vi "main.vi"() -> ()   [LabVIEW 2022 SP3]
uses:
  <vilib>/express/express arith-compare/Formula/XNode/ExpressFormulaBlockNode.xnode
panel:
  in  "Día":i32=1 min=1 max=365
  out "Dia_a":i32
  out "Diciembre":bool
  out "Noviembre":bool
  out "Octubre":bool
  out "Septiembre":bool
  out "Agosto":bool
  out "Julio":bool
  out "Junio":bool
  out "Mayo":bool
  out "Abril":bool
  out "Marzo":bool
  out "Febrero":bool
  out "Enero":bool
  in  "Stop Button":bool
  in  "Manual - Automático":bool
  out "Ángulo":dbl
  out "Altitud":dbl
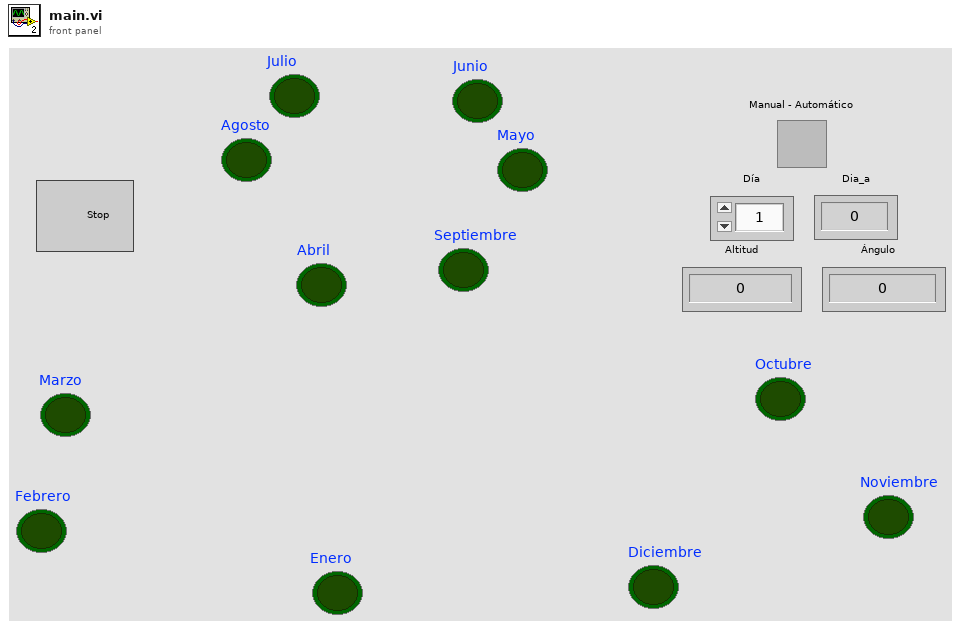
[diagram p1: front panel]
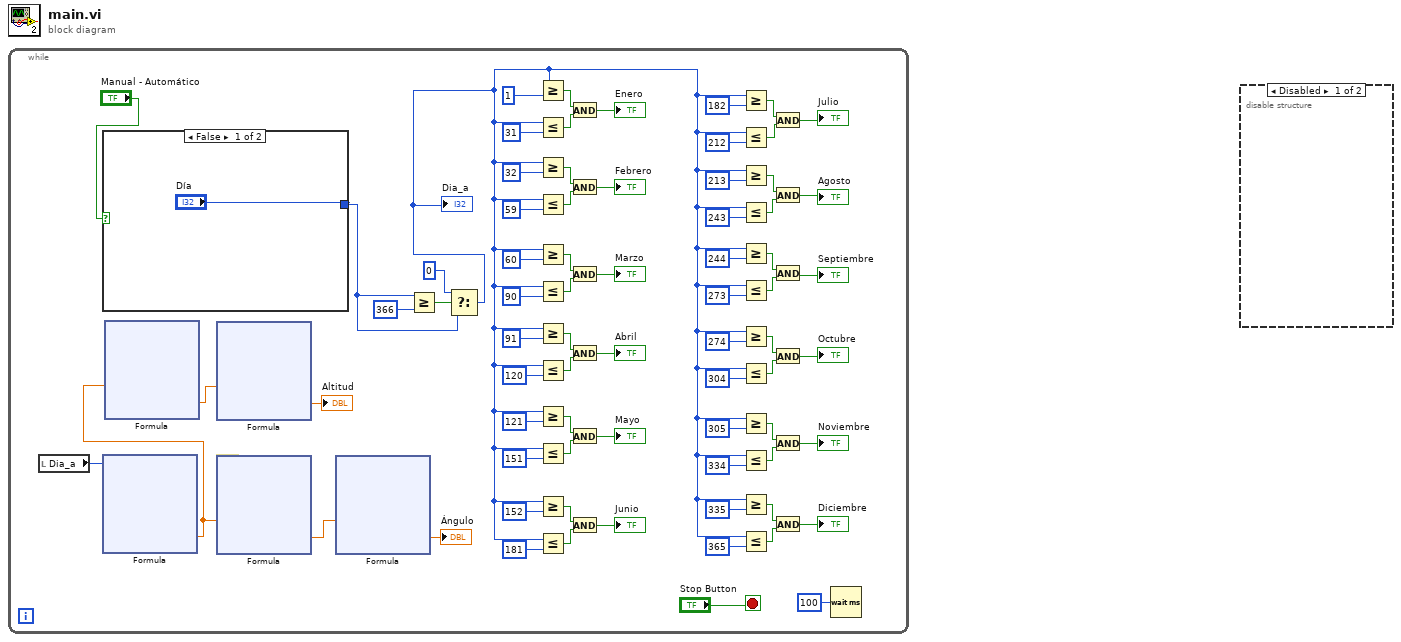
[diagram p0: block diagram]
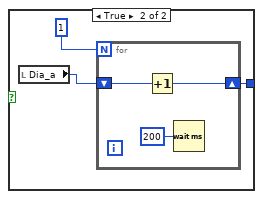
[diagram p3: hidden frame]
diagram:
  n1 = while {
    stop <- "Stop Button" stop-if-true
    # "Altitud"
    # "dx"
    # "x"
    # "Angulo"
    # "f(x)"
    n2 = local read "Dia_a"() -> (w6:i32)
    n3 = case shown="False" "Manual - Automático" {
      tunnel: ["Día" w117] -> w1
      frame False {
      }
      frame True {
        n4 = local read "Dia_a"() -> (w116:i32)
        n5 = for {
          N: 1 -> [_]
          shift-right: [w119] -> w117
          shift-left: w116 -> [w120]
          n6 = Increment(x=w120) -> (x+1=w119:i32)
          n7 = Wait (ms)(milliseconds to wait=u32 200) -> ()  [unwired: 1 out]
        }
      }
    }
    n8 = xnode "Formula"("dia"=w6) -> ("Result"=w9:dbl)  [unwired: 1 in, 1 out]
    n9 = xnode "Formula"("X"=w9) -> ("Result"=w8:dbl)  [unwired: 1 in, 1 out]
    n10 = xnode "Formula"("dx"=w8) -> ("Result"=→"Altitud":dbl)  [unwired: 1 in, 1 out]
    n11 = xnode "Formula"("X"=w9) -> ("Result"=w11:dbl)  [unwired: 1 in, 1 out]
    n12 = xnode "Formula"("fx"=w11) -> ("Result"=→"Ángulo":dbl)  [unwired: 1 in, 1 out]
    n13 = Greater Or Equal?(x=w1, y=366) -> (x >= y?=w4:bool)
    n14 = Select(t=0 ("f"), s=w4, f=w1) -> (s? t:f=w3:i32)
    "Dia_a" <- w3
    n15 = Greater Or Equal?(x=w3, y=1) -> (x >= y?=w73:bool)
    n16 = Less Or Equal?(x=w3, y=31) -> (x <= y?=w72:bool)
    n17 = Greater Or Equal?(x=w3, y=32) -> (x >= y?=w69:bool)
    n18 = Less Or Equal?(x=w3, y=59) -> (x <= y?=w68:bool)
    n19 = Greater Or Equal?(x=w3, y=60) -> (x >= y?=w62:bool)
    n20 = Less Or Equal?(x=w3, y=90) -> (x <= y?=w63:bool)
    n21 = Greater Or Equal?(x=w3, y=91) -> (x >= y?=w61:bool)
    n22 = Less Or Equal?(x=w3, y=120) -> (x <= y?=w60:bool)
    n23 = Greater Or Equal?(x=w3, y=121) -> (x >= y?=w57:bool)
    n24 = Less Or Equal?(x=w3, y=151) -> (x <= y?=w56:bool)
    n25 = Greater Or Equal?(x=w3, y=152) -> (x >= y?=w51:bool)
    n26 = Less Or Equal?(x=w3, y=181) -> (x <= y?=w52:bool)
    n27 = And(x=w73, y=w72) -> (x .and. y?=→"Enero":bool)
    n28 = And(x=w69, y=w68) -> (x .and. y?=→"Febrero":bool)
    n29 = And(x=w62, y=w63) -> (x .and. y?=→"Marzo":bool)
    n30 = And(x=w61, y=w60) -> (x .and. y?=→"Abril":bool)
    n31 = And(x=w57, y=w56) -> (x .and. y?=→"Mayo":bool)
    n32 = And(x=w51, y=w52) -> (x .and. y?=→"Junio":bool)
    n33 = Greater Or Equal?(x=w3, y=182) -> (x >= y?=w50:bool)
    n34 = Less Or Equal?(x=w3, y=212) -> (x <= y?=w49:bool)
    n35 = Greater Or Equal?(x=w3, y=213) -> (x >= y?=w46:bool)
    n36 = Less Or Equal?(x=w3, y=243) -> (x <= y?=w45:bool)
    n37 = Greater Or Equal?(x=w3, y=244) -> (x >= y?=w42:bool)
    n38 = Less Or Equal?(x=w3, y=273) -> (x <= y?=w41:bool)
    n39 = Greater Or Equal?(x=w3, y=274) -> (x >= y?=w38:bool)
    n40 = Less Or Equal?(x=w3, y=304) -> (x <= y?=w37:bool)
    n41 = Greater Or Equal?(x=w3, y=305) -> (x >= y?=w34:bool)
    n42 = Less Or Equal?(x=w3, y=334) -> (x <= y?=w33:bool)
    n43 = Greater Or Equal?(x=w3, y=335) -> (x >= y?=w30:bool)
    n44 = Less Or Equal?(x=w3, y=365) -> (x <= y?=w29:bool)
    n45 = And(x=w50, y=w49) -> (x .and. y?=→"Julio":bool)
    n46 = And(x=w46, y=w45) -> (x .and. y?=→"Agosto":bool)
    n47 = And(x=w42, y=w41) -> (x .and. y?=→"Septiembre":bool)
    n48 = And(x=w38, y=w37) -> (x .and. y?=→"Octubre":bool)
    n49 = And(x=w34, y=w33) -> (x .and. y?=→"Noviembre":bool)
    n50 = And(x=w30, y=w29) -> (x .and. y?=→"Diciembre":bool)
    n51 = Wait (ms)(milliseconds to wait=u32 100) -> ()  [unwired: 1 out]
  }
  n52 = disable-structure shown="Disabled" {
    frame Disabled {
    }
    frame Enabled {
    }
  }
